vi "ISTEQ TroSpec.vi"() -> ()   [LabVIEW 2015]
doc: "Example VI that demonstrates all library features."
uses:
  PL ISTEQ TroSpec.lvclass
  <vilib>/Analysis/baseanly.llb/Mean (DBL).vi
  <vilib>/Analysis/NI_AALBase.lvlib
panel:
  in  "save configuration":bool
  out "lost frames":u16
  out "acquisition in progress":bool
  in  "acquisition":bool
  out "graph":u32[](graph)
  in  "configuration":T1 {"gain" items=["1", "3", "5", "7"]; "period, s" format="%#_6p"}
  out "device information":T2 {"max period, s" format="%#_6p"; "min period, s" format="%#_6p"; "CCD type" items=["Toshiba TCD1304AP"=1, "Hamamatsu G11620-512DA"=2, "Hamamatsu 3901-512Q"=3]}
  out "TroSpec":refnum<class "PL ISTEQ TroSpec.lvclass">
  in  "product id":u16=35254 format="%04x"
  in  "vendor id":u16=1240 format="%04x"
  out "error":errorcluster
  in  "stop":bool
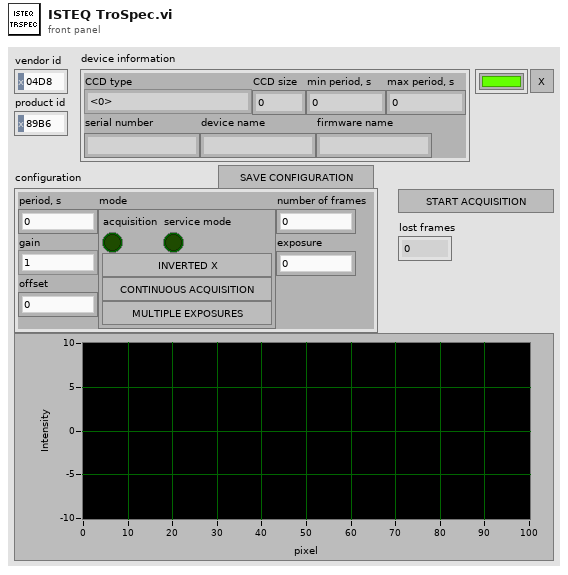
[diagram p1: front panel]
types:
  T1 = cluster{"period, s":dbl, "gain":u16, "offset":u16, "mode":cluster{"acquisition":bool, "service mode":bool, "inverted X":bool, "continuous acquisition":bool, "multiple exposures":bool}, "number of frames":u32, "exposure":u32}
  T2 = cluster{"CCD type":u16, "CCD size":u16, "min period, s":dbl, "max period, s":dbl, "serial number":string, "device name":string, "firmware name":string}
  T3 = cluster{"inverted X":bool, "continuous acquisition":bool, "multiple exposures":bool}
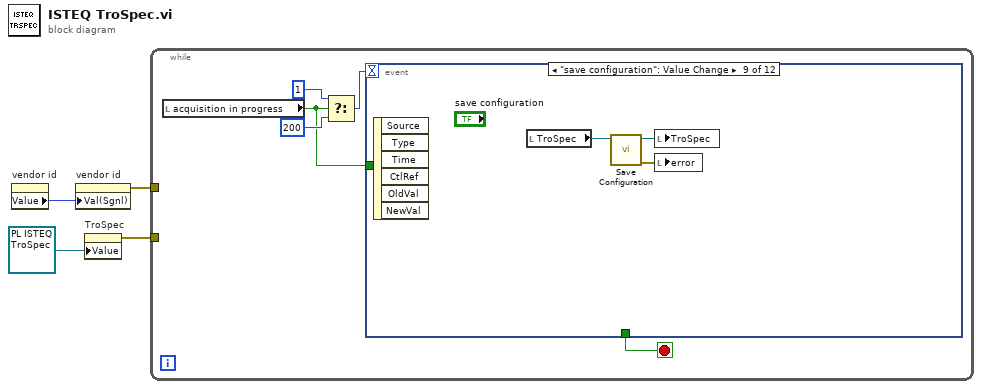
[diagram p0: block diagram]
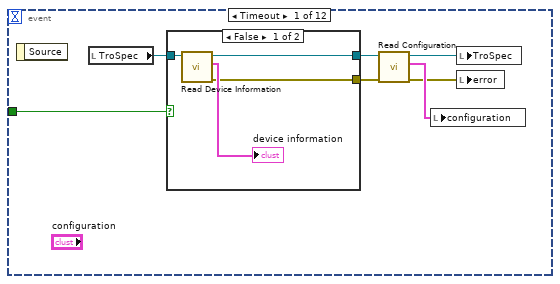
[diagram p2: hidden frame]
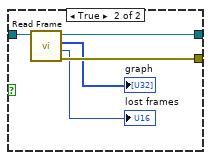
[diagram p3: hidden frame]
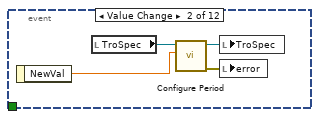
[diagram p4: hidden frame]
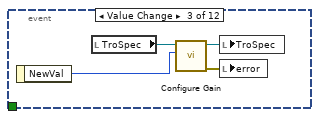
[diagram p5: hidden frame]
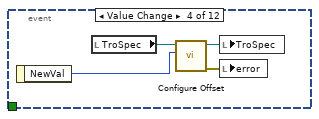
[diagram p6: hidden frame]
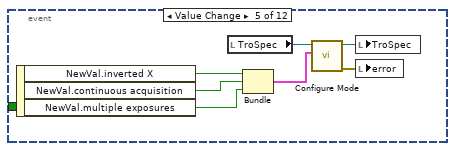
[diagram p7: hidden frame]
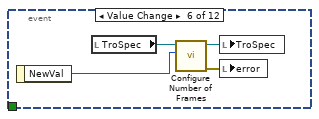
[diagram p8: hidden frame]
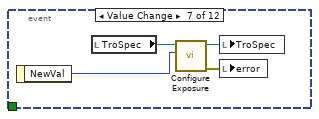
[diagram p9: hidden frame]
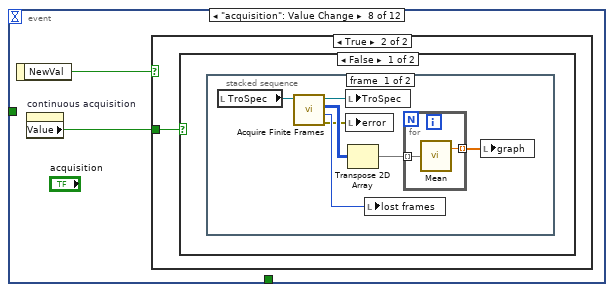
[diagram p10: hidden frame]
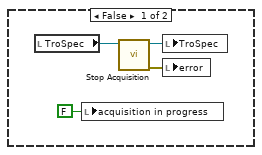
[diagram p11: hidden frame]
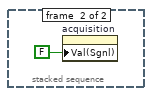
[diagram p12: hidden frame]
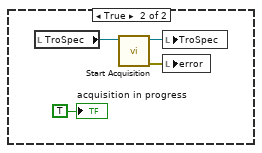
[diagram p13: hidden frame]
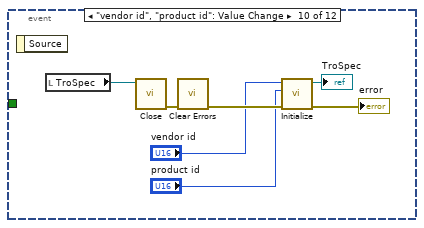
[diagram p14: hidden frame]
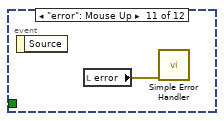
[diagram p15: hidden frame]
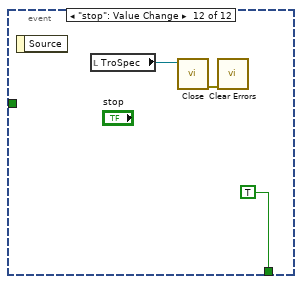
[diagram p16: hidden frame]
diagram:
  n1 = property on="vendor id" class="DigNum (strict)"() -> ("Value"=w4:u16)  [unwired: 2 in, 2 out]
  n2 = property on="vendor id" class="DigNum (strict)"("Val(Sgnl)"=w4) -> (error out=w3:errorcluster)  [unwired: 2 in, 1 out]
  n3 = property on="TroSpec" class="LVClassControl (strict)"("Value"=refnum<class "PL ISTEQ TroSpec.lvclass"> refnum ("PL ISTEQ TroSpec.lvclass")) -> (error out=w1:errorcluster)  [unwired: 2 in, 1 out]
  n4 = while {
    tunnel: w3 -> [_]
    tunnel: w1 -> [_]
    stop <- w9 stop-if-true
    n5 = local read "acquisition in progress"() -> (w5:bool)
    n6 = Select(t=1, s=w5, f=200) -> (s? t:f=w6:i32)
    n7 = event shown="[8] \"save configuration\": Value Change" {
      selector: _ -> [_ _ _ _ _ _ _ _ _ _ _ _]
      dyn-events: _ -> [_ _ _ _ _ _ _ _ _ _ _ _]
      timeout: w6 -> [_ _ _ _ _ _ _ _ _ _ _ _]
      tunnel: [_ _ _ _ _ _ _ _ _ _ _ TRUE ("stop")] -> w9
      tunnel: w5 -> [w15 _ _ _ _ _ _ _ _ _ _ _]
      event Timeout {
        n8 = event-data() -> ()  [unwired: 1 in, 1 out]
        n9 = local read "TroSpec"() -> (w16:refnum<class "PL ISTEQ TroSpec.lvclass">)
        n10 = case shown="False" w15 {
          tunnel: w16 -> [w20 w25]
          tunnel: [w17 w23] -> w11
          tunnel: [w18 w24] -> w12
          frame False {
            n11 = call "Read Device Information.vi"("TroSpec in"=w20) -> ("error out"=w17:errorcluster, "device information"=→"device information":T2, "TroSpec out"=w18:refnum<class "PL ISTEQ TroSpec.lvclass">)  [unwired: 8 in]
          }
          frame True {
            n12 = call "Read Frame.vi"("TroSpec in"=w25) -> ("error out"=w23:errorcluster, "lost frames"=→"lost frames":u16, "frame"=→"graph":u32[], "TroSpec out"=w24:refnum<class "PL ISTEQ TroSpec.lvclass">)  [unwired: 7 in]
          }
        }
        n13 = call "Read Configuration.vi"("error in (no error)"=w11, "TroSpec in"=w12) -> ("error out"=w10:errorcluster, "configuration"=w14:T1, "TroSpec out"=w13:refnum<class "PL ISTEQ TroSpec.lvclass">)  [unwired: 7 in]
        n14 = local write "configuration"(w14) -> ()
        n15 = local write "TroSpec"(w13) -> ()
        n16 = local write "error"(w10) -> ()
      }
      event "configuration.period, s": Value Change {
        n17 = event-data() -> ("NewVal"=w26:dbl)  [unwired: 1 in]
        n18 = local read "TroSpec"() -> (w29:refnum<class "PL ISTEQ TroSpec.lvclass">)
        n19 = call "Configure Period.vi"("period, s"=w26, "TroSpec in"=w29) -> ("error out"=w27:errorcluster, "TroSpec out"=w28:refnum<class "PL ISTEQ TroSpec.lvclass">)  [unwired: 8 in]
        n20 = local write "TroSpec"(w28) -> ()
        n21 = local write "error"(w27) -> ()
      }
      event "configuration.gain": Value Change {
        n22 = event-data() -> ("NewVal"=w30:u16)  [unwired: 1 in]
        n23 = local read "TroSpec"() -> (w33:refnum<class "PL ISTEQ TroSpec.lvclass">)
        n24 = call "Configure Gain.vi"("gain"=w30, "TroSpec in"=w33) -> ("error out"=w31:errorcluster, "TroSpec out"=w32:refnum<class "PL ISTEQ TroSpec.lvclass">)  [unwired: 8 in]
        n25 = local write "TroSpec"(w32) -> ()
        n26 = local write "error"(w31) -> ()
      }
      event "configuration.offset": Value Change {
        n27 = event-data() -> ("NewVal"=w34:u16)  [unwired: 1 in]
        n28 = local read "TroSpec"() -> (w37:refnum<class "PL ISTEQ TroSpec.lvclass">)
        n29 = call "Configure Offset.vi"("offset"=w34, "TroSpec in"=w37) -> ("error out"=w35:errorcluster, "TroSpec out"=w36:refnum<class "PL ISTEQ TroSpec.lvclass">)  [unwired: 8 in]
        n30 = local write "TroSpec"(w36) -> ()
        n31 = local write "error"(w35) -> ()
      }
      event "configuration.mode": Value Change {
        n32 = event-data() -> ("NewVal.inverted X"=w41:bool, "NewVal.continuous acquisition"=w40:bool, "NewVal.multiple exposures"=w39:bool)  [unwired: 1 in]
        n33 = local read "TroSpec"() -> (w44:refnum<class "PL ISTEQ TroSpec.lvclass">)
        n34 = Bundle("inverted X"=w41, "continuous acquisition"=w40, "multiple exposures"=w39) -> (w38:T3)  [unwired: 1 in]
        n35 = call "Configure Mode.vi"("mode"=w38, "TroSpec in"=w44) -> ("error out"=w42:errorcluster, "TroSpec out"=w43:refnum<class "PL ISTEQ TroSpec.lvclass">)  [unwired: 8 in]
        n36 = local write "TroSpec"(w43) -> ()
        n37 = local write "error"(w42) -> ()
      }
      event "configuration.number of frames": Value Change {
        n38 = event-data() -> ("NewVal"=w45:u32)  [unwired: 1 in]
        n39 = local read "TroSpec"() -> (w48:refnum<class "PL ISTEQ TroSpec.lvclass">)
        n40 = call "Configure Number of Frames.vi"("number of frames"=w45, "TroSpec in"=w48) -> ("error out"=w46:errorcluster, "TroSpec out"=w47:refnum<class "PL ISTEQ TroSpec.lvclass">)  [unwired: 8 in]
        n41 = local write "TroSpec"(w47) -> ()
        n42 = local write "error"(w46) -> ()
      }
      event "configuration.exposure": Value Change {
        n43 = event-data() -> ("NewVal"=w49:u32)  [unwired: 1 in]
        n44 = local read "TroSpec"() -> (w52:refnum<class "PL ISTEQ TroSpec.lvclass">)
        n45 = call "Configure Exposure.vi"("exposure"=w49, "TroSpec in"=w52) -> ("error out"=w50:errorcluster, "TroSpec out"=w51:refnum<class "PL ISTEQ TroSpec.lvclass">)  [unwired: 8 in]
        n46 = local write "TroSpec"(w51) -> ()
        n47 = local write "error"(w50) -> ()
      }
      event "acquisition": Value Change {
        n48 = event-data() -> ("NewVal"=w54:bool)  [unwired: 1 in]
        n49 = property on="continuous acquisition" class="Bool (strict)"() -> ("Value"=w53:bool)  [unwired: 2 in, 2 out]
        n50 = case shown="True" w54 {
          tunnel: w53 -> [_ w59]
          frame False {
            n51 = local read "TroSpec"() -> (w56:refnum<class "PL ISTEQ TroSpec.lvclass">)
            n52 = local write "acquisition in progress"(FALSE ("acquisition in progress")) -> ()
            n53 = call "Stop Acquisition.vi"("TroSpec in"=w56) -> ("error out"=w58:errorcluster, "TroSpec out"=w57:refnum<class "PL ISTEQ TroSpec.lvclass">)  [unwired: 9 in]
            n54 = local write "TroSpec"(w57) -> ()
            n55 = local write "error"(w58) -> ()
          }
          frame True {
            n56 = case shown="False" w59 {
              frame False {
                n57 = stacked-sequence {
                  frame #0 {
                    n58 = local read "TroSpec"() -> (w60:refnum<class "PL ISTEQ TroSpec.lvclass">)
                    n59 = call "Acquire Finite Frames.vi"("TroSpec in"=w60) -> ("error out"=w62:errorcluster, "lost frames"=w63:u16, "frame"=w64:u32[][], "TroSpec out"=w61:refnum<class "PL ISTEQ TroSpec.lvclass">)  [unwired: 7 in]
                    n60 = local write "TroSpec"(w61) -> ()
                    n61 = local write "error"(w62) -> ()
                    n62 = Transpose 2D Array(2D array=w64) -> (transposed array=w65:u32[][])
                    n63 = local write "lost frames"(w63) -> ()
                    n64 = for {
                      tunnel: w65 -> [w67] mode=indexing
                      tunnel: [w68] -> w66 mode=indexing
                      n65 = call-poly <vilib>:"Mean.vi"("X"=w67) -> ("mean"=w68:dbl)  [unwired: 1 out]
                    }
                    n66 = local write "graph"(w66) -> ()
                  }
                  frame #1 {
                    n67 = property on="acquisition" class="Bool (strict)"("Val(Sgnl)"=FALSE ("acquisition")) -> ()  [unwired: 2 in, 2 out]
                  }
                }
              }
              frame True {
                n68 = local read "TroSpec"() -> (w71:refnum<class "PL ISTEQ TroSpec.lvclass">)
                n69 = call "Start Acquisition.vi"("TroSpec in"=w71) -> ("error out"=w73:errorcluster, "TroSpec out"=w72:refnum<class "PL ISTEQ TroSpec.lvclass">)  [unwired: 9 in]
                n70 = local write "TroSpec"(w72) -> ()
                n71 = local write "error"(w73) -> ()
                "acquisition in progress" <- TRUE ("acquisition in progress")
              }
            }
          }
        }
      }
      event "save configuration": Value Change {
        n72 = event-data() -> ()  [unwired: 1 in, 6 out]
        n73 = local read "TroSpec"() -> (w76:refnum<class "PL ISTEQ TroSpec.lvclass">)
        n74 = call "Save Configuration.vi"("TroSpec in"=w76) -> ("error out"=w74:errorcluster, "TroSpec out"=w75:refnum<class "PL ISTEQ TroSpec.lvclass">)  [unwired: 9 in]
        n75 = local write "TroSpec"(w75) -> ()
        n76 = local write "error"(w74) -> ()
      }
      event "vendor id", "product id": Value Change {
        n77 = event-data() -> ()  [unwired: 1 in, 1 out]
        n78 = local read "TroSpec"() -> (w79:refnum<class "PL ISTEQ TroSpec.lvclass">)
        n79 = call "Close.vi"("TroSpec in"=w79) -> ("error out"=w82:errorcluster)  [unwired: 10 in]
        n80 = call <vilib>:"Clear Errors.vi"("error in (no error)"=w82) -> ("error out"=w81:errorcluster)  [unwired: 5 in, 1 out]
        n81 = call "Initialize.vi"("error in (no error)"=w81, "product id (0x89B6)"="product id", "vendor id (0x04D8)"="vendor id") -> ("error out"=→"error":errorcluster, "TroSpec out"=→"TroSpec":refnum<class "PL ISTEQ TroSpec.lvclass">)  [unwired: 7 in]
      }
      event "error": Mouse Up {
        n82 = event-data() -> ()  [unwired: 1 in, 1 out]
        n83 = local read "error"() -> (w84:errorcluster)
        n84 = call <vilib>:"Simple Error Handler.vi"("error in (no error)"=w84) -> ()  [unwired: 4 in, 5 out]
      }
      event "stop": Value Change {
        n85 = event-data() -> ()  [unwired: 1 in, 1 out]
        n86 = local read "TroSpec"() -> (w85:refnum<class "PL ISTEQ TroSpec.lvclass">)
        n87 = call "Close.vi"("TroSpec in"=w85) -> ("error out"=w86:errorcluster)  [unwired: 10 in]
        n88 = call <vilib>:"Clear Errors.vi"("error in (no error)"=w86) -> ()  [unwired: 5 in, 2 out]
      }
    }
  }
